vi "Get version and date for EXE.vi"(11 "error out":errorcluster) -> (3 "Version":i32, 4 "Build date":string, 6 "Stable Version?":bool, 8 "Development Version?":bool, 15 "error out":errorcluster)   [LabVIEW 2013]
uses:
  <vilib>/Utility/config.llb/Read Key (Boolean).vi
  <vilib>/Utility/config.llb/Read Key (Double).vi
  <vilib>/Utility/config.llb/Read Key (I32).vi
  <vilib>/Utility/config.llb/NI_LVConfig.lvlib
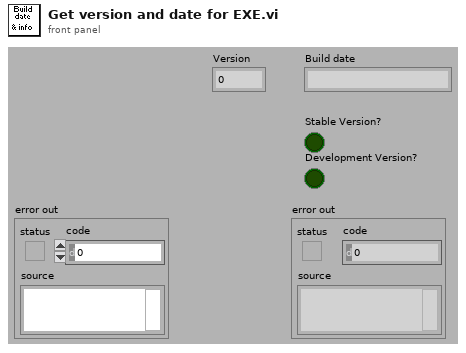
[diagram p1: front panel]
types:
  T1 = typedef "NI_LVConfig.lvlib/Config Data RefNum.ctl" = refnum<k1>
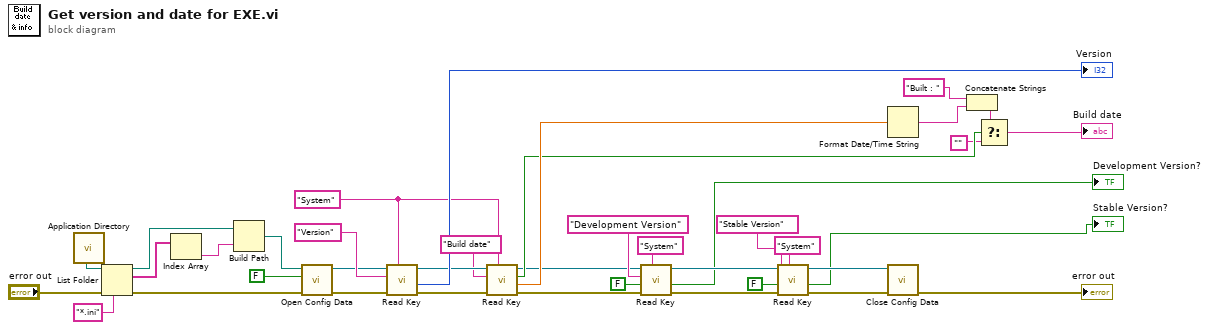
[diagram p0: block diagram]
diagram:
  w22 = "System" ("section")
  n1 = call <vilib>:"Application Directory.vi"() -> ("Application Directory"=w30:path)
  n2 = List Folder(path=w30, pattern="*.ini", error in="error out") -> (path out=w34:path, filenames=w27:string[], error out=w35:errorcluster)  [unwired: 1 in, 1 out]
  n3 = Index Array(array=w27) -> (element=w33:string)  [unwired: 1 in]
  n4 = Build Path(base path=w34, name or relative path=w33) -> (appended path=w32:path)
  n5 = call <vilib>:"Open Config Data.vi"("error in (no error)"=w35, "create file if necessary (T)"=FALSE, "configuration file path"=w32) -> ("error out"=w28:errorcluster, "refnum"=w29:T1)  [unwired: 6 in, 1 out]
  n6 = call-poly <vilib>:"Read Key.vi"("section"=w22, "error in (no error)"=w28, "key"="Version" ("section"), "refnum"=w29) -> ("error out"=w24:errorcluster, "value"=→"Version":i32, "refnum out"=w25:T1)  [unwired: 4 in, 1 out]
  n7 = call-poly <vilib>:"Read Key.vi"("section"=w22, "error in (no error)"=w24, "key"="Build date", "refnum"=w25) -> ("error out"=w7:errorcluster, "value"=w21:dbl, "found?"=w20:bool, "refnum out"=w8:T1)  [unwired: 4 in]
  n8 = call-poly <vilib>:"Read Key.vi"("section"="System", "error in (no error)"=w7, "default value"=FALSE, "key"="Development Version", "refnum"=w8) -> ("error out"=w10:errorcluster, "value"=→"Development Version?":bool, "refnum out"=w9:T1)  [unwired: 3 in, 1 out]
  n9 = call-poly <vilib>:"Read Key.vi"("section"="System", "error in (no error)"=w10, "default value"=FALSE, "key"="Stable Version", "refnum"=w9) -> ("error out"=w5:errorcluster, "value"=→"Stable Version?":bool, "refnum out"=w6:T1)  [unwired: 3 in, 1 out]
  n10 = Format Date/Time String(seconds (now)=w21) -> (date/time string=w17:string)  [unwired: 2 in]
  n11 = call <vilib>:"Close Config Data.vi"("error in (no error)"=w5, "refnum"=w6) -> ("error out"=→"error out":errorcluster)  [unwired: 8 in, 1 out]
  n12 = Concatenate Strings("Built : " ("string"), w17) -> (w16:string)
  n13 = Select(t=w16, s=w20, f="") -> (s? t:f=→"Build date":string)
